vi "UIRef.vi"(8 "error in":errorcluster, 11 "cDAQ in":refnum<class "PLTarget cDAQ.lvclass">) -> (0 "error out":errorcluster, 2 "VI refnum":refnum<vi>, 3 "cDAQ out":refnum<class "PLTarget cDAQ.lvclass">)   [LabVIEW 2013, in "PLTarget cDAQ.lvclass"]
uses:
  PLTarget cDAQ.lvclass
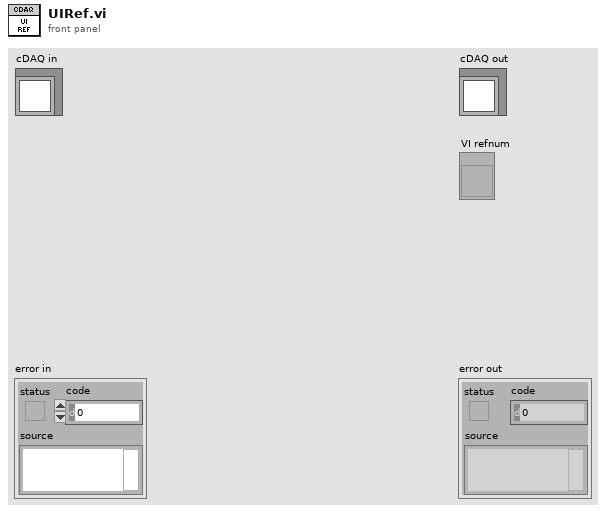
[diagram p1: front panel]
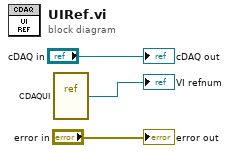
[diagram p0: block diagram]
diagram:
  n1 = vi-ref "CDAQUI.vi"() -> (→"VI refnum":refnum<vi>)
  "error out" <- "error in"
  "cDAQ out" <- "cDAQ in"
